vi "PCO_SetDelayExposureTime.vi"(4 "wTimebaseExposure":enum16{"ns", "µs", "ms"}(ring), 6 "wTimebaseDelay":enum16{"ns", "µs", "ms"}(ring), 8 "error in (no error)":errorcluster, 9 "dwExposure":u32, 10 "dwDelay":u32, 11 "Handle":u64) -> (0 "error out":errorcluster, 3 "Handle Out":u64, 5 "return type":u32 format="%x")   [LabVIEW 2011]
uses:
  SC2_Cam64.dll
panel:
  # "A00A3002 invalid Handle"
  # "schön, geht auch asynchron!"
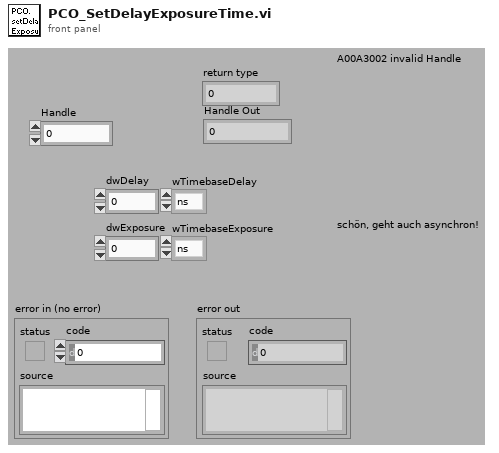
[diagram p1: front panel]
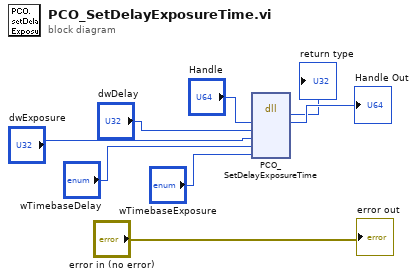
[diagram p0: block diagram]
diagram:
  n1 = dll-call lib="C:/Program Files/colibri/Drivers/PCO.Camera/SC2_Cam*.*" fn="PCO_SetDelayExposureTime"("Handle"="Handle", "dwDelay"="dwDelay", "dwExposure"="dwExposure", "wTimeBaseDelay"="wTimebaseDelay", "wTimeBaseExposure"="wTimebaseExposure") -> ("return type"=→"return type":u32, "Handle"=→"Handle Out":u64)  [unwired: 5 in, 4 out]
  "error out" <- "error in (no error)"
